vi "Emitter-Count-FFT_lfTester.vi"(4 "Bar Image Path":path, 5 "Error In":errorcluster, 6 "Emitter #":i32=27, 7 "Threshold (%)":dbl(slide)=20.0 min=0.0 max=100.0 step=1.0 scale=0.0..100.0 scale format="%#.1f") -> (0 "Error Out":errorcluster, 1 "Fit Profile":dbl[][](graph), 2 "Emitter Intensity":dbl[](array[numeric])=[0.024052367008515582, 0.024378595803643897, 0.025805706649686327, 0.041269063644883704, 0.37978020475060875, 0.8269249741034874, 0.5506416954032008, 0.2766134312094456, 0.5222093424752133, 0.6745161500069505, 0.3837297031878495, 0.45121422133334527, 0.7103637619224853, 0.716317717698865, 0.7171865400913889, 0.7369553324394739, 0.7848537912046026, 0.7350321520338291, 0.8064454289852603, 0.7830645776065793, 0.7315417281381865, 0.746674372093649, 0.8191162226517132, 0.8872941171195007, 0.9241792711308816, 1.0] format="%#_3g", 3 "Emitter Count":i32=23)   [LabVIEW 2017]
uses:
  <vilib>/Analysis/2dsp.llb/Real FFT.vi
  <vilib>/Analysis/NI_AALPro.lvlib
panel:
  in  "Optional Rectangle":i32[](array[numeric])=[100, 1131, 2511, 1331]
  out "Best Fit Offset":i32=22
  in  "Optimization":T1(ring)=enum."3-Point Quadratic Fit"
  in  "Zero Padding":bool=TRUE
  out "Best Fit Pitch":dbl=81.40903944063709 format="%#.1f"
  # "Emitter Count Calculation Based on Fourier Transform"
  # "Author: Yufeng Li\nModified by Chao Gong"
  # "Best Fit Result"
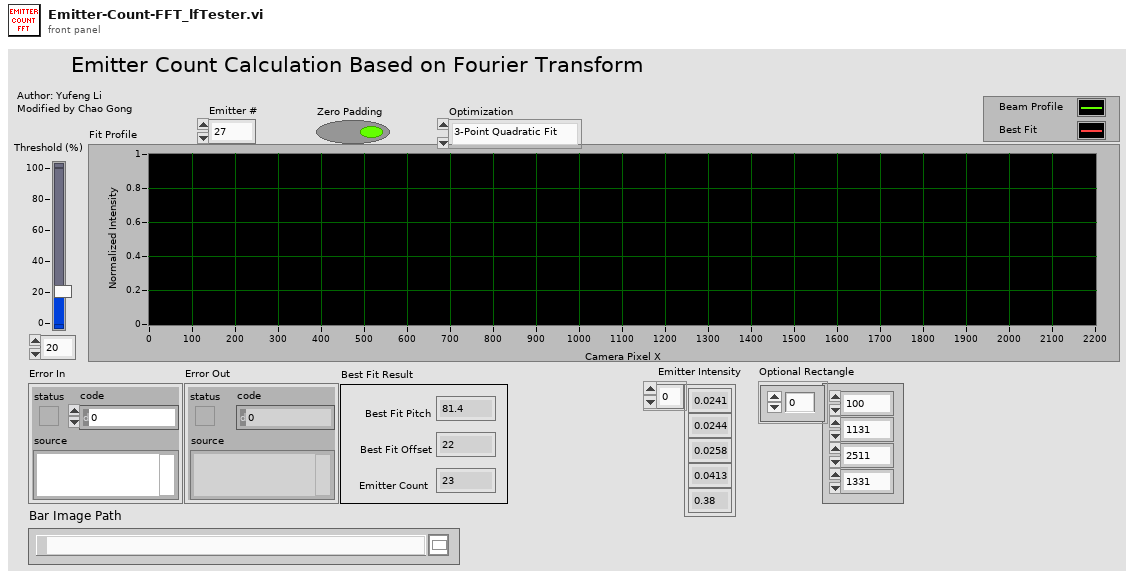
[diagram p1: front panel]
types:
  T1 = enum16{"None", "3-Point Quadratic Fit", "5-Point Quadratic Fit", "5-Point Gaussian Fit"}
  T2 = enum16{"Init", "Fit Pitch", "Fit Offset", "Emitter Calc", "Done"}
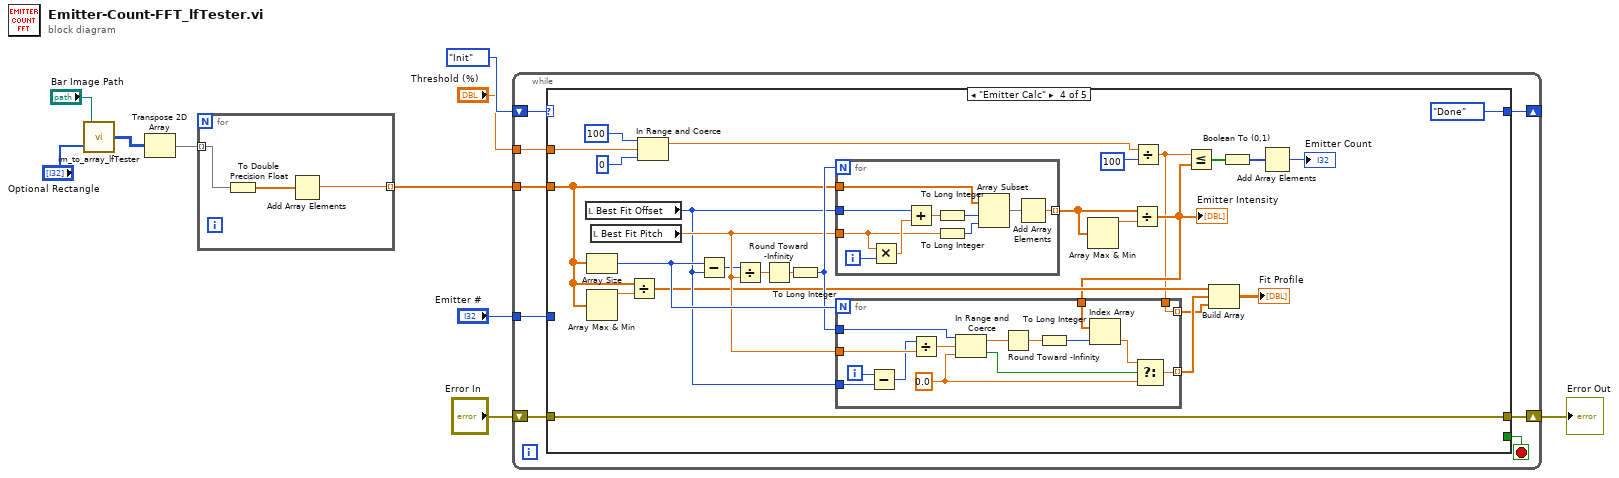
[diagram p0: block diagram]
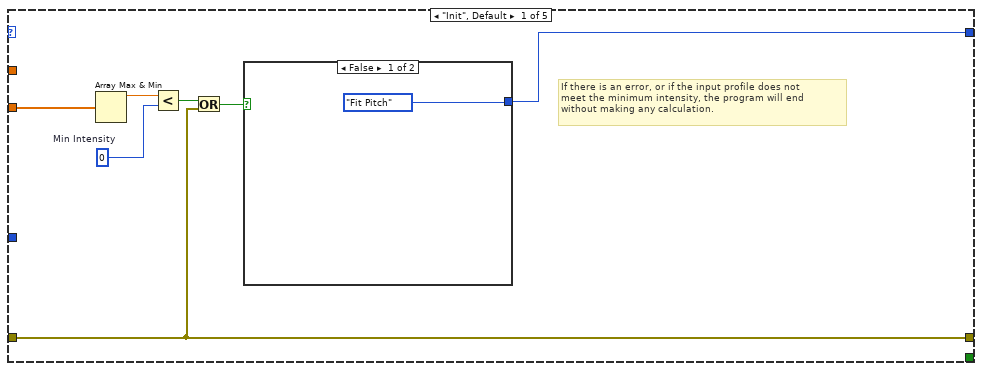
[diagram p2: hidden frame]
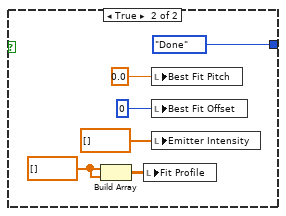
[diagram p3: hidden frame]
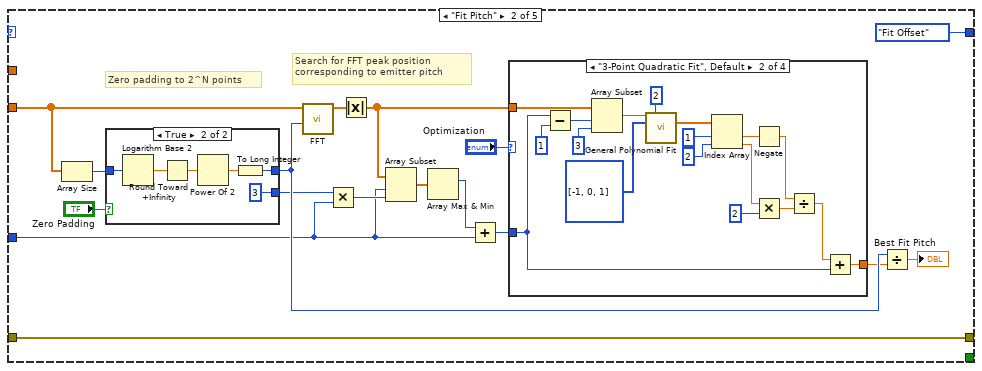
[diagram p4: hidden frame]
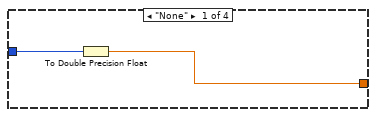
[diagram p5: hidden frame]
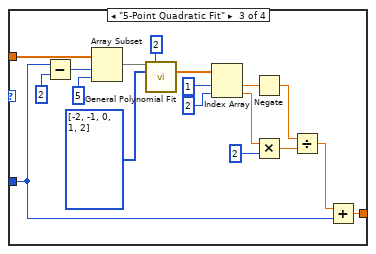
[diagram p6: hidden frame]
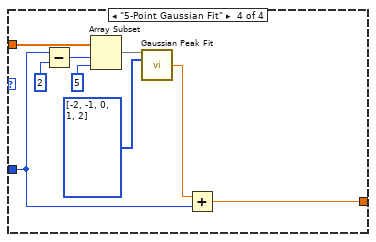
[diagram p7: hidden frame]
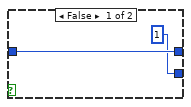
[diagram p8: hidden frame]
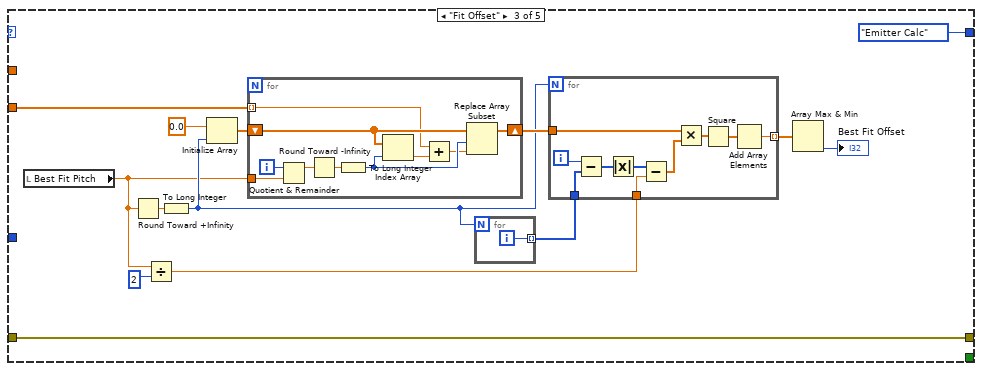
[diagram p9: hidden frame]
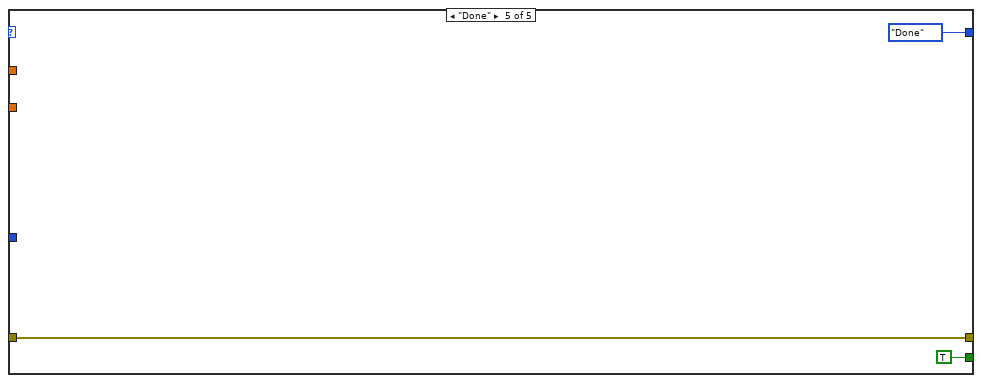
[diagram p10: hidden frame]
diagram:
  n1 = call "im_to_array_lfTester.vi"("Optional Rectangle"="Optional Rectangle", "Image file path"="Bar Image Path") -> ("Pixels Values"=w4:u8[][])
  n2 = Transpose 2D Array(2D array=w4) -> (transposed array=w3:u8[][])
  n3 = for {
    tunnel: w3 -> [w12] mode=indexing
    tunnel: [w13] -> w2 mode=indexing
    n4 = To Double Precision Float(number=w12) -> (double precision float=w11:dbl[])
    n5 = Add Array Elements(numeric array=w11) -> (sum=w13:dbl)
  }
  n6 = while {
    tunnel: w2 -> [w20]
    shift-right: [w18] -> w9
    shift-left: "Error In" -> [w19]
    tunnel: "Emitter #" -> [w15]
    shift-right: [w17] -> _
    shift-left: T2."Init" ("Sequence") -> [w21]
    tunnel: "Threshold (%)" -> [w14]
    stop <- w16 stop-if-true
    n7 = case shown="\"Emitter Calc\"" w21 {
      tunnel: w20 -> [w24 w40 w116 w156 _]
      tunnel: w19 -> [w23 w36 w115 w155 w196]
      tunnel: [w23 w36 w115 w155 w196] -> w18
      tunnel: [w22 T2."Fit Offset" ("Sequence") T2."Emitter Calc" ("Sequence") T2."Done" ("Sequence") T2."Done" ("Sequence")] -> w17
      tunnel: [_ _ _ _ TRUE] -> w16
      tunnel: w15 -> [_ w38 _ _ _]
      tunnel: w14 -> [_ _ _ w148 _]
      frame "Init", Default {
        w26 = 0  # Min Intensity
        # "If there is an error, or if the input profile does not \nmeet the minimum intensity, the program will end \nwithout making any calculation."
        n8 = Array Max & Min(array=w24) -> (max value=w25:dbl)  [unwired: 3 out]
        n9 = Less?(x=w25, y=w26) -> (x < y?=w27:bool)
        n10 = Or(x=w27, y=w23) -> (x .or. y?=w28:bool)
        n11 = case shown="False" w28 {
          tunnel: [T2."Fit Pitch" ("Sequence") T2."Done" ("Sequence")] -> w22
          frame False {
          }
          frame True {
            w32 = dbl[] []
            n12 = Build Array(w32, w32) -> (w30:dbl[][])
            n13 = local write "Fit Profile"(w30) -> ()
            n14 = local write "Best Fit Pitch"(0.0) -> ()
            n15 = local write "Best Fit Offset"(0) -> ()
            n16 = local write "Emitter Intensity"(dbl[] []) -> ()
          }
        }
      }
      frame "Fit Pitch" {
        # "Search for FFT peak position\ncorresponding to emitter pitch"
        # "Zero padding to 2^N points"
        n17 = Array Size(array=w40) -> (size(s)=w41:i32)
        n18 = case shown="True" "Zero Padding" {
          tunnel: w41 -> [w101 w107]
          tunnel: [w101 w103] -> w50
          tunnel: [1 3] -> w42
          frame False {
          }
          frame True {
            n19 = Logarithm Base 2(1:w107) -> (0:w106:dbl)
            n20 = Round Toward +Infinity(x=w106) -> (ceil(x): smallest int >= x=w105:dbl)
            n21 = Power Of 2(x=w105) -> (2^x=w104:dbl)
            n22 = To Long Integer(number=w104) -> (32bit integer=w103:i32)
          }
        }
        n23 = call-poly <vilib>:"FFT.vi"("FFT size"=w50, "X"=w40) -> ("FFT {X}"=w46:cdb[])  [unwired: 8 in, 1 out]
        n24 = Multiply(x=w42, y=w38) -> (x*y=w44:i32)
        n25 = Absolute Value(x=w46) -> (abs(x)=w48:dbl[])
        n26 = Array Subset(array=w48, index=w38, length=w44) -> (w43:dbl[])
        n27 = Array Max & Min(array=w43) -> (max index (indices)=w45:i32)  [unwired: 3 out]
        n28 = Add(x=w45, y=w38) -> (x+y=w49:i32)
        n29 = case shown="\"3-Point Quadratic Fit\", Default" "Optimization" {
          tunnel: w48 -> [_ w57 w77 w93]
          tunnel: w49 -> [w54 w56 w76 w92]
          tunnel: [w53 w55 w73 w91] -> w47
          frame "None" {
            n30 = To Double Precision Float(number=w54) -> (double precision float=w53:dbl)
          }
          frame "3-Point Quadratic Fit", Default {
            n31 = Subtract(x=w56, y=1) -> (x-y=w62:i32)
            n32 = Array Subset(array=w57, index=w62, length=3) -> (w59:dbl[])
            n33 = call <vilib>:"General Polynomial Fit.vi"("Y"=w59, "polynomial order"=2, "X"=i32[] [-1, 0, 1]) -> ("Polynomial Coefficients"=w64:dbl[])  [unwired: 9 in, 3 out]
            n34 = Index Array(array=w64, index #1=1, index #2=2) -> (element #1=w71:dbl, element #2=w68:dbl)
            n35 = Negate(x=w71) -> (-x=w72:dbl)
            n36 = Multiply(x=w68, y=2) -> (x*y=w69:dbl)
            n37 = Divide(x=w72, y=w69) -> (x/y=w70:dbl)
            n38 = Add(x=w70, y=w56) -> (x+y=w55:dbl)
          }
          frame "5-Point Quadratic Fit" {
            n39 = Subtract(x=w76, y=2) -> (x-y=w80:i32)
            n40 = Array Subset(array=w77, index=w80, length=5) -> (w75:dbl[])
            n41 = call <vilib>:"General Polynomial Fit.vi"("Y"=w75, "polynomial order"=2, "X"=i32[] [-2, -1, 0, 1, 2]) -> ("Polynomial Coefficients"=w82:dbl[])  [unwired: 9 in, 3 out]
            n42 = Index Array(array=w82, index #1=1, index #2=2) -> (element #1=w89:dbl, element #2=w86:dbl)
            n43 = Negate(x=w89) -> (-x=w90:dbl)
            n44 = Multiply(x=w86, y=2) -> (x*y=w87:dbl)
            n45 = Divide(x=w90, y=w87) -> (x/y=w88:dbl)
            n46 = Add(x=w88, y=w76) -> (x+y=w73:dbl)
          }
          frame "5-Point Gaussian Fit" {
            n47 = Subtract(x=w92, y=2) -> (x-y=w96:i32)
            n48 = Array Subset(array=w93, index=w96, length=5) -> (w98:dbl[])
            n49 = call <vilib>:"Gaussian Peak Fit.vi"("Y"=w98, "X"=i32[] [-2, -1, 0, 1, 2]) -> ("center"=w97:dbl)  [unwired: 7 in, 6 out]
            n50 = Add(x=w97, y=w92) -> (x+y=w91:dbl)
          }
        }
        n51 = Divide(x=w50, y=w47) -> (x/y=→"Best Fit Pitch":dbl)
      }
      frame "Fit Offset" {
        n52 = local read "Best Fit Pitch"() -> (w111:dbl)
        n53 = Round Toward +Infinity(x=w111) -> (ceil(x): smallest int >= x=w117:dbl)
        n54 = Divide(x=w111, y=2) -> (x/y=w110:dbl)
        n55 = To Long Integer(number=w117) -> (32bit integer=w113:i32)
        n56 = Initialize Array(0.0 ("element"), w113) -> (w120:dbl[])
        n57 = for {
          tunnel: w116 -> [w135] mode=indexing
          shift-right: [w141] -> w118
          shift-left: w120 -> [w142]
          tunnel: w111 -> [w139]
          i -> [w140]
          n58 = Quotient & Remainder(x=w140, y=w139) -> (x-y*floor(x/y)=w137:dbl)  [unwired: 1 out]
          n59 = Round Toward -Infinity(1:w137) -> (0:w138:dbl)
          n60 = To Long Integer(number=w138) -> (32bit integer=w134:i32)
          n61 = Index Array(array=w142, index=w134) -> (element=w136:dbl)
          n62 = Add(x=w135, y=w136) -> (x+y=w133:dbl)
          n63 = Replace Array Subset(array=w142, new element=w133, index=w134) -> (w141:dbl[])
        }
        n64 = for {
          N: w113 -> [_]
          tunnel: [w122] -> w108 mode=indexing
          i -> [w122]
        }
        n65 = for {
          N: w113 -> [_]
          tunnel: w118 -> [w130]
          tunnel: [w132] -> w119 mode=indexing
          tunnel: w110 -> [w124]
          tunnel: w108 -> [w123]
          i -> [w129]
          n66 = Subtract(x=w129, y=w123) -> (x-y=w131:i32[])
          n67 = Absolute Value(x=w131) -> (abs(x)=w125:i32[])
          n68 = Subtract(x=w125, y=w124) -> (x-y=w126:dbl[])
          n69 = Multiply(x=w130, y=w126) -> (x*y=w128:dbl[])
          n70 = Square(x=w128) -> (x^2=w127:dbl[])
          n71 = Add Array Elements(numeric array=w127) -> (sum=w132:dbl)
        }
        n72 = Array Max & Min(array=w119) -> (min index (indices)=→"Best Fit Offset":i32)  [unwired: 3 out]
      }
      frame "Emitter Calc" {
        n73 = local read "Best Fit Offset"() -> (w166:i32)
        n74 = Array Size(array=w156) -> (size(s)=w169:i32)
        n75 = Array Max & Min(array=w156) -> (max value=w163:dbl)  [unwired: 3 out]
        n76 = local read "Best Fit Pitch"() -> (w167:dbl)
        n77 = Divide(x=w156, y=w163) -> (x/y=w164:dbl[])
        n78 = In Range and Coerce(upper limit=100, x=w148, lower limit=0) -> (coerced(x)=w144:dbl)  [unwired: 1 out]
        n79 = Subtract(x=w169, y=w166) -> (x-y=w157:i32)
        n80 = Divide(x=w157, y=w167) -> (x/y=w159:dbl)
        n81 = Round Toward -Infinity(1:w159) -> (0:w158:dbl)
        n82 = To Long Integer(number=w158) -> (32bit integer=w168:i32)
        n83 = for {
          N: w168 -> [_]
          tunnel: w167 -> [w189]
          tunnel: w166 -> [w192]
          tunnel: w156 -> [w186]
          tunnel: [w185] -> w161 mode=indexing
          i -> [w194]
          n84 = Multiply(x=w189, y=w194) -> (x*y=w193:dbl)
          n85 = Add(x=w192, y=w193) -> (x+y=w191:dbl)
          n86 = To Long Integer(number=w191) -> (32bit integer=w190:i32)
          n87 = To Long Integer(number=w189) -> (32bit integer=w188:i32)
          n88 = Array Subset(array=w186, index=w190, length=w188) -> (w187:dbl[])
          n89 = Add Array Elements(numeric array=w187) -> (sum=w185:dbl)
        }
        n90 = Array Max & Min(array=w161) -> (max value=w160:dbl)  [unwired: 3 out]
        n91 = Divide(x=w161, y=w160) -> (x/y=w152:dbl[])
        "Emitter Intensity" <- w152
        n92 = Divide(x=w144, y=100) -> (x/y=w143:dbl)
        n93 = for {
          N: w169 -> [_]
          tunnel: w167 -> [w184]
          tunnel: w166 -> [w182]
          tunnel: w168 -> [w171]
          tunnel: w152 -> [w176]
          tunnel: [w172] -> w162 mode=indexing
          tunnel: [w170] -> w145 mode=indexing
          tunnel: w143 -> [w170]
          i -> [w183]
          w173 = 0.0 ("element")
          n94 = Subtract(x=w183, y=w182) -> (x-y=w181:i32)
          n95 = Divide(x=w181, y=w184) -> (x/y=w180:dbl)
          n96 = In Range and Coerce(upper limit=w171, x=w180, lower limit=w173) -> (coerced(x)=w179:dbl, In Range?=w174:bool)
          n97 = Round Toward -Infinity(1:w179) -> (0:w177:dbl)
          n98 = To Long Integer(number=w177) -> (32bit integer=w178:i32)
          n99 = Index Array(array=w176, index=w178) -> (element=w175:dbl)
          n100 = Select(t=w175, s=w174, f=w173) -> (s? t:f=w172:dbl)
        }
        n101 = Less Or Equal?(x=w143, y=w152) -> (x <= y?=w151:bool[])
        n102 = Build Array(w164, w162, w145) -> (→"Fit Profile":dbl[][])
        n103 = Boolean To (0,1)(Boolean=w151) -> (0, 1=w150:i16[])
        n104 = Add Array Elements(numeric array=w150) -> (sum=→"Emitter Count":i16)
      }
      frame "Done" {
      }
    }
  }
  "Error Out" <- w9
